vi "calculate z.vi"(0 "Z":T1 {"zm" format="%.8f"; "zt" format="%.8f"; "zi" format="%.8f"}, 7 "Chi_A":dbl format="%#_13g", 11 "T [K]":dbl format="%#_13g") -> (8 "Z":dbl format="%#_13g")   [LabVIEW 2017, in "LicorLI7000.lvlib"]
uses:
  LicorLI7000.lvlib
  Z parameter.ctl
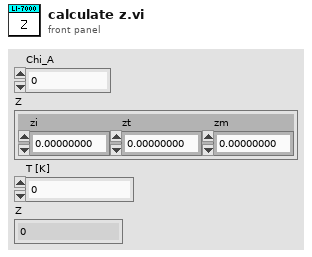
[diagram p1: front panel]
types:
  T1 = typedef "LicorLI7000.lvlib/Z parameter.ctl" = cluster{"zi":dbl, "zt":dbl, "zm":dbl}
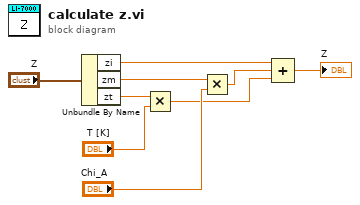
[diagram p0: block diagram]
diagram:
  n1 = Unbundle By Name("Z") -> ("zi"=w7:dbl, "zm"=w8:dbl, "zt"=w5:dbl)
  n2 = Multiply(x=w5, y="T [K]") -> (x*y=w2:dbl)
  n3 = Multiply(x=w8, y="Chi_A") -> (x*y=w3:dbl)
  n4 = Compound Arithmetic op=ADD(w7, w3, w2) -> (→"Z":dbl)
